vi "TDMS Path.vi"(8 "error in":errorcluster, 10 "Socket":string="0", 11 "Sequence Context In":refnum<k7>) -> (0 "error out":errorcluster, 3 "File path":path=path "C:/Rawlogfiles/DUT/2022Jul31/092816_")   [LabVIEW 2021]
uses:
  <vilib>/addons/TestStand/_TSUtility.llb/TestStand - Get Property Value (String).vi
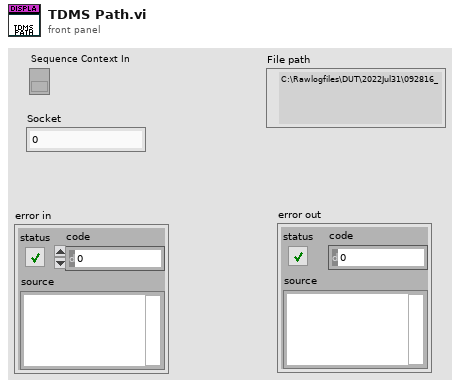
[diagram p1: front panel]
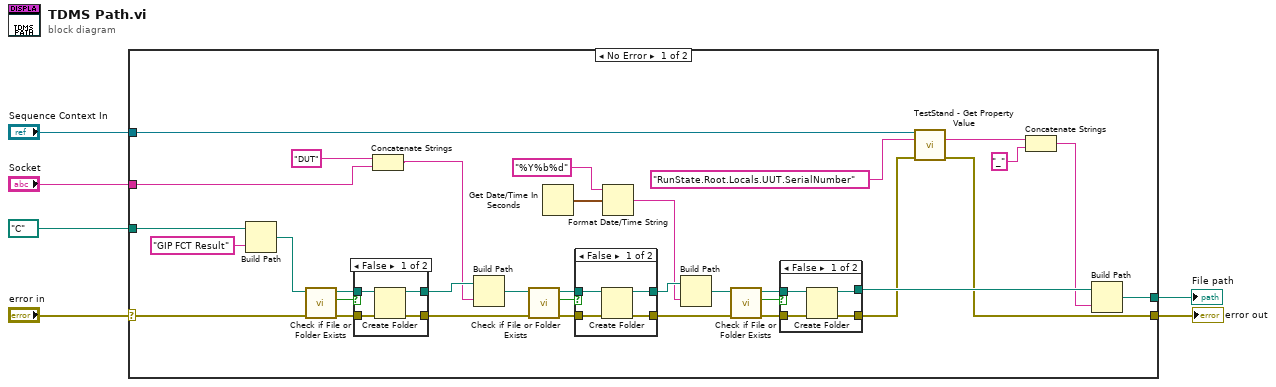
[diagram p0: block diagram]
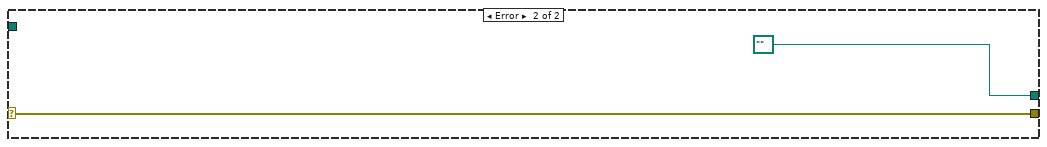
[diagram p5: hidden frame]
diagram:
  n1 = case shown="No Error" "error in" {
    selector: "error in" -> [w34 w60]
    tunnel: [w9 w60] -> w5
    tunnel: "Socket" -> [w13 _]
    tunnel: path "C:/" ("Application Directory") -> [w33 _]
    tunnel: [w17 path "" ("appended path")] -> w3
    tunnel: "Sequence Context In" -> [w11 _]
    frame No Error {
      n2 = Build Path(base path=w33, name or relative path="GIP FCT Result" ("relative uri")) -> (appended path=w35:path)
      n3 = call <vilib>:"Check if File or Folder Exists.vi"("error in (no error)"=w34, "path"=w35) -> ("error out"=w37:errorcluster, "file or folder exists?"=w38:bool, "dup path"=w36:path)  [unwired: 7 in]
      n4 = case shown="False" w38 {
        tunnel: w37 -> [w56 w58]
        tunnel: [w55 w58] -> w22
        tunnel: w36 -> [w54 w57]
        tunnel: [w53 w57] -> w40
        frame False {
          n5 = Create Folder(path (use dialog)=w54, error in=w56) -> (created path=w53:path, error out=w55:errorcluster)  [unwired: 1 in, 1 out]
        }
        frame True {
        }
      }
      n6 = Concatenate Strings("DUT" ("string"), w13) -> (w12:string)
      n7 = Build Path(base path=w40, name or relative path=w12) -> (appended path=w29:path)
      n8 = call <vilib>:"Check if File or Folder Exists.vi"("error in (no error)"=w22, "path"=w29) -> ("error out"=w32:errorcluster, "file or folder exists?"=w30:bool, "dup path"=w31:path)  [unwired: 7 in]
      n9 = Get Date/Time In Seconds() -> (seconds since 1Jan1904=w21:timestamp)
      n10 = case shown="False" w30 {
        tunnel: w32 -> [w50 w52]
        tunnel: [w49 w52] -> w23
        tunnel: w31 -> [w48 w51]
        tunnel: [w47 w51] -> w28
        frame False {
          n11 = Create Folder(path (use dialog)=w48, error in=w50) -> (created path=w47:path, error out=w49:errorcluster)  [unwired: 1 in, 1 out]
        }
        frame True {
        }
      }
      n12 = Format Date/Time String(time format string (%c)="%Y%b%d", seconds (now)=w21) -> (date/time string=w19:string)  [unwired: 1 in]
      n13 = Build Path(base path=w28, name or relative path=w19) -> (appended path=w24:path)
      n14 = call <vilib>:"Check if File or Folder Exists.vi"("error in (no error)"=w23, "path"=w24) -> ("error out"=w25:errorcluster, "file or folder exists?"=w27:bool, "dup path"=w26:path)  [unwired: 7 in]
      n15 = case shown="False" w27 {
        tunnel: w25 -> [w44 w46]
        tunnel: [w43 w46] -> w10
        tunnel: w26 -> [w42 w45]
        tunnel: [w41 w45] -> w18
        frame False {
          n16 = Create Folder(path (use dialog)=w42, error in=w44) -> (created path=w41:path, error out=w43:errorcluster)  [unwired: 1 in, 1 out]
        }
        frame True {
        }
      }
      n17 = call-poly <vilib>:"TestStand - Get Property Value.vi"("Sequence Context In"=w11, "Lookup String"="RunState.Root.Locals.UUT.SerialNumber", "error in (no error)"=w10) -> ("Value"=w8:string, "error out"=w9:errorcluster)  [unwired: 10 in, 1 out]
      n18 = Concatenate Strings(w8, "_" ("regular expression")) -> (w16:string)
      n19 = Build Path(base path=w18, name or relative path=w16) -> (appended path=w17:path)
    }
    frame Error {
    }
  }
  "error out" <- w5
  "File path" <- w3
